vi "inject.vi"(1 "volume":i32) -> ()   [LabVIEW 2023]
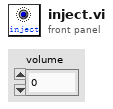
[diagram p1: front panel]
types:
  T1 = enum16{"plate1", "plate2", "plate3", "rinse", "seat"}
  T2 = enum16{"Initialize", "Absolute Position", "Relative Pickup", "Relative Dispense", "Swich valve", "Bypass"}
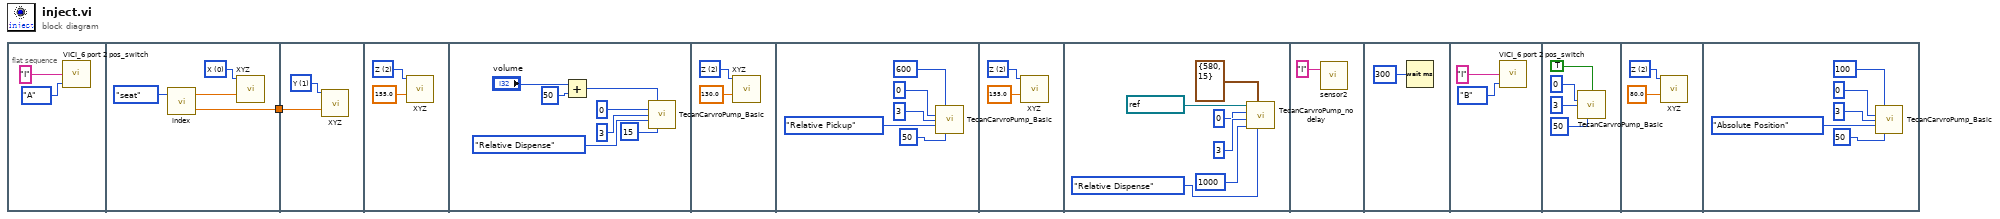
[diagram p0: block diagram]
diagram:
  n1 = flat-sequence {
    tunnel: [w4] -> w1
    tunnel: w1 -> [w8]
    frame #0 {
      n2 = call "VICI_6 port 2 pos_switch.vi"("Switch to position (A/B)"=enum16{"A", "B"}."A", "Valve ID"="I") -> ()  [unwired: 2 in, 1 out]
    }
    frame #1 {
      w7 = u16 0 items=["X", "Y", "Z"] ("AXIS")
      n3 = call "index.vi"("where"=T1."seat") -> ("Y"=w4:dbl, "X"=w5:dbl)  [unwired: 1 in]
      n4 = call "XYZ.vi"("AXIS"=w7, "Set location (mm)"=w5) -> ()  [unwired: 9 in, 5 out]
    }
    frame #2 {
      w9 = u16 1 items=["X", "Y", "Z"] ("AXIS")
      n5 = call "XYZ.vi"("AXIS"=w9, "Set location (mm)"=w8) -> ()  [unwired: 9 in, 5 out]
    }
    frame #3 {
      w11 = u16 2 items=["X", "Y", "Z"] ("AXIS")
      n6 = call "XYZ.vi"("AXIS"=w11, "Set location (mm)"=155.0) -> ()  [unwired: 9 in, 5 out]
    }
    frame #4 {
      n7 = Add(x="volume", y=50) -> (x+y=w17:i32)
      n8 = call "TecanCarvroPump_Basic.vi"("Volume (μL)"=w17, "TecanPump address"=u8 0, "Valve"=u8 3, "Mode"=T2."Relative Dispense", "Speed (μL/s)"=u16 15) -> ()  [unwired: 10 in, 1 out]
    }
    frame #5 {
      w20 = u16 2 items=["X", "Y", "Z"] ("AXIS")
      n9 = call "XYZ.vi"("AXIS"=w20, "Set location (mm)"=130.0) -> ()  [unwired: 9 in, 5 out]
    }
    frame #6 {
      n10 = call "TecanCarvroPump_Basic.vi"("Volume (μL)"=u16 600, "TecanPump address"=u8 0, "Valve"=u8 3, "Mode"=T2."Relative Pickup", "Speed (μL/s)"=u16 50) -> ()  [unwired: 10 in, 1 out]
    }
    frame #7 {
      w27 = u16 2 items=["X", "Y", "Z"] ("AXIS")
      n11 = call "XYZ.vi"("AXIS"=w27, "Set location (mm)"=155.0) -> ()  [unwired: 9 in, 5 out]
    }
    frame #8 {
      n12 = call "TecanCarvroPump_no delay.vi"("Mode"=T2."Relative Dispense", "TecanPump parameters"=cluster{"Volume (μL)":u16, "Speed (μL/s)":u16} {"Volume (μL)"=580, "Speed (μL/s)"=15}, "Syringe size (μL)"=u16 1000, "Valve"=u8 3, "TecanPump address"=u8 0, "TecanPump COM"=refnum<visa-resource-name> "COM6") -> ()  [unwired: 1 out]
    }
    frame #9 {
      n13 = call "sensor2.vi"("Sensor"="I") -> ()  [unwired: 1 in, 2 out]
    }
    frame #10 {
      n14 = Wait (ms)(milliseconds to wait=u32 300) -> ()  [unwired: 1 out]
    }
    frame #11 {
      n15 = call "VICI_6 port 2 pos_switch.vi"("Switch to position (A/B)"=enum16{"A", "B"}."B", "Valve ID"="I") -> ()  [unwired: 2 in, 1 out]
    }
    frame #12 {
      n16 = call "TecanCarvroPump_Basic.vi"("急停"=TRUE, "TecanPump address"=u8 0, "Valve"=u8 3, "Speed (μL/s)"=u16 50) -> ()  [unwired: 11 in, 1 out]
    }
    frame #13 {
      w43 = u16 2 items=["X", "Y", "Z"] ("AXIS")
      n17 = call "XYZ.vi"("AXIS"=w43, "Set location (mm)"=80.0) -> ()  [unwired: 9 in, 5 out]
    }
    frame #14 {
      n18 = call "TecanCarvroPump_Basic.vi"("Volume (μL)"=u16 100, "TecanPump address"=u8 0, "Valve"=u8 3, "Mode"=T2."Absolute Position", "Speed (μL/s)"=u16 50) -> ()  [unwired: 10 in, 1 out]
    }
  }
